vi "Update Value.vi"(6 "Time":dbl, 8 "error in (no error)":errorcluster, 11 "DblNumericStatusIndicator in":refnum<class "DblNumericStatusIndicator.lvclass">) -> (0 "error out":errorcluster, 1 "Update":bool, 2 "Value":variant, 3 "DblNumericStatusIndicator out":refnum<class "DblNumericStatusIndicator.lvclass">)   [LabVIEW 2020, in "VolatusGUI.lvlib" / "DblNumericStatusIndicator.lvclass"]
uses:
  DblNumericStatusIndicator.lvclass
  DblNumericStatusIndicator.lvclass/DblNumericStatusIndicator.ctl
  lv-vecto/Vecto/Channel/Channel.lvclass
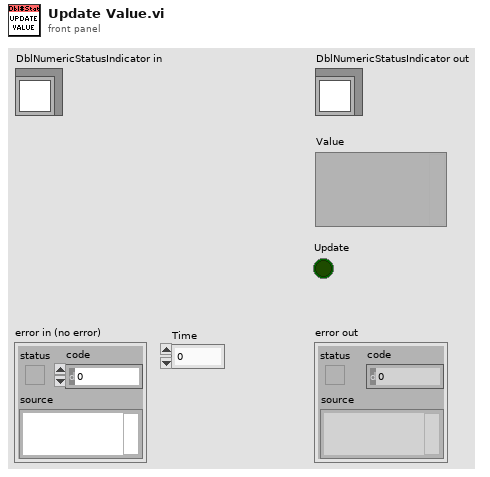
[diagram p1: front panel]
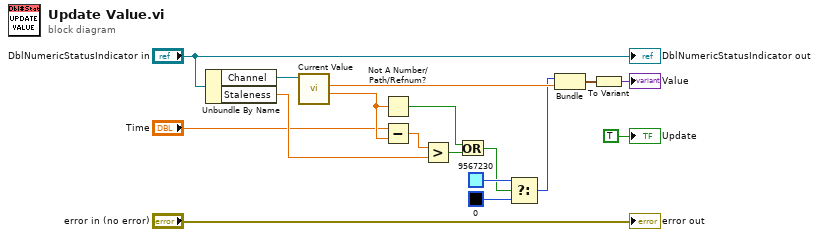
[diagram p0: block diagram]
diagram:
  n1 = Unbundle By Name("DblNumericStatusIndicator in") -> ("Channel"=w16:refnum<class "Channel.lvclass">, "Staleness"=w6:dbl)
  n2 = call "Current Value.vi"("Channel in"=w16) -> ("Timestamp"=w5:dbl, "Scaled"=w14:dbl)  [unwired: 6 in, 3 out]
  n3 = Not A Number/Path/Refnum?(number/path/refnum=w5) -> (NaN/Path/Refnum?=w3:bool)
  n4 = Subtract(x="Time", y=w5) -> (x-y=w7:dbl)
  n5 = Greater?(x=w7, y=w6) -> (0:w11:bool)
  n6 = Or(x=w3, y=w11) -> (x .or. y?=w4:bool)
  n7 = Select(t=u32 9567230, s=w4, f=u32 0) -> (s? t:f=w10:u32)
  n8 = Bundle(w10, "Scaled"=w14) -> (w9:cluster{u32, "Scaled":dbl})  [unwired: 1 in]
  n9 = To Variant(anything=w9) -> (Variant=→"Value":variant)
  "error out" <- "error in (no error)"
  "DblNumericStatusIndicator out" <- "DblNumericStatusIndicator in"
  "Update" <- TRUE ("Update")
